vi "Get Group ID.vi"(11 "Transfer Group Timing in":refnum<class "Transfer Group Timing.lvclass">) -> (2 "Group ID":i32, 3 "Transfer Group Timing out":refnum<class "Transfer Group Timing.lvclass">)   [LabVIEW 2017, in "DSF Core.lvlib" / "Transfer Group Timing.lvclass"]
uses:
  Transfer Group Timing.lvclass
  Transfer Group Timing.lvclass/Transfer Group Timing.ctl
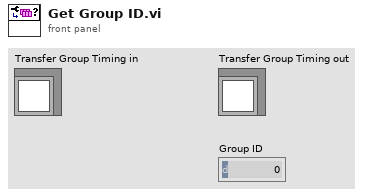
[diagram p1: front panel]
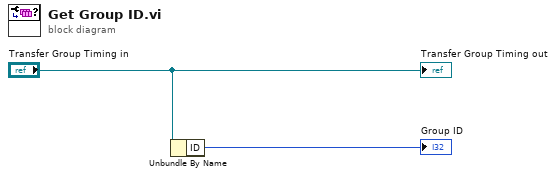
[diagram p0: block diagram]
diagram:
  n1 = Unbundle By Name("Transfer Group Timing in") -> ("ID"=→"Group ID":i32)
  "Transfer Group Timing out" <- "Transfer Group Timing in"
